vi "3ph Power 1Hz to Summary FileS.vi"(7 "1Hz Filename":string, 9 "3ph sample rate [Hz]":dbl, 10 "3phf samples per channel":i32, 11 "Queue in":refnum<queue>) -> ()   [LabVIEW 2019]
uses:
  Globals and Definitions/Initialization Globals.vi
  Globals and Definitions/RT Globals RD v1.0.vi
  <vilib>/Utility/file.llb/Write Delimited Spreadsheet (string).vi
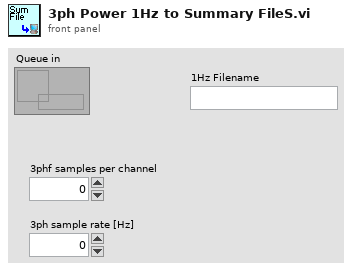
[diagram p1: front panel]
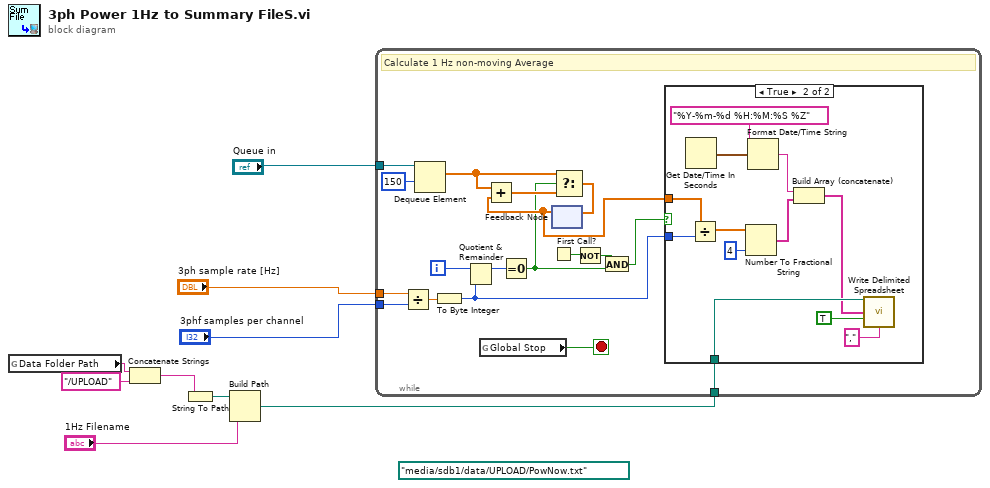
[diagram p0: block diagram]
diagram:
  (unwired) path "/media/sdb1/data/UPLOAD/PowNow.txt" ("file path")
  n1 = global read "Initialization Globals.vi" "Data Folder Path"() -> (w4:string)
  n2 = Concatenate Strings(w4, "/UPLOAD" ("string")) -> (w2:string)
  n3 = String To Path(string=w2) -> (path=w7:path)
  n4 = Build Path(base path=w7, name or relative path="1Hz Filename") -> (appended path=w6:path)
  n5 = while {
    tunnel: "3phf samples per channel" -> [w21]
    tunnel: "3ph sample rate [Hz]" -> [w22]
    tunnel: w6 -> [w18]
    tunnel: "Queue in" -> [w12]
    i -> [w27]
    stop <- w13 stop-if-true
    # "Calculate 1 Hz non-moving Average"
    n6 = Divide(x=w22, y=w21) -> (x/y=w20:dbl)
    n7 = Dequeue Element(queue=w12, timeout in ms (-1)=150) -> (element=w11:dbl[])  [unwired: 1 in, 3 out]
    n8 = To Byte Integer(number=w20) -> (8bit integer=w19:i8)
    n9 = Quotient & Remainder(x=w27, y=w19) -> (x-y*floor(x/y)=w26:i32)  [unwired: 1 out]
    n10 = global read "RT Globals RD v1.0.vi" "Global Stop"() -> (w13:bool)
    n11 = Equal To 0?(x=w26) -> (x = 0?=w17:bool)
    n12 = First Call?() -> (First Call?: T/F=w15:bool)
    n13 = feedback #1() -> (w23:dbl[])  [unwired: 1 in]
    n14 = Add(x=w11, y=w23) -> (x+y=w25:dbl[])
    n15 = Select(t=w11, s=w17, f=w25) -> (s? t:f=w24:dbl[])
    n16 = feedback-in #1(w24) -> ()
    n17 = Not(x=w15) -> (.not. x?=w14:bool)
    n18 = And(x=w14, y=w17) -> (x .and. y?=w16:bool)
    n19 = case shown="True" w16 {
      tunnel: w23 -> [_ w39]
      tunnel: w19 -> [_ w38]
      tunnel: w18 -> [_ w29]
      frame False {
      }
      frame True {
        n20 = Get Date/Time In Seconds() -> (seconds since 1Jan1904=w36:timestamp)
        n21 = Divide(x=w39, y=w38) -> (x/y=w34:dbl[])
        n22 = Number To Fractional String(number=w34, precision (6)=i16 4) -> (F-format string=w32:string[])  [unwired: 2 in]
        n23 = Format Date/Time String(time format string (%c)="%Y-%m-%d %H:%M:%S %Z", seconds (now)=w36) -> (date/time string=w33:string)  [unwired: 1 in]
        n24 = Build Array (concatenate)(w33, w32) -> (w28:string[])
        n25 = call-poly <vilib>:"Write Delimited Spreadsheet.vi"("file path (dialog if empty)"=w29, "1D data"=w28, "append to file? (new file:F)"=TRUE, "delimiter (\\t)"="," ("delimiter (\\t)")) -> ()  [unwired: 10 in, 2 out]
      }
    }
  }
